vi "Camera To Target Grid.vi"(2 "Height":dbl format="%#_13g", 3 "Width":dbl format="%#_13g", 4 "CY":dbl format="%#_13g", 5 "CX":dbl format="%#_13g") -> (0 "Y'":dbl format="%#_13g", 1 "X'":dbl format="%#_13g")   [LabVIEW 2013]
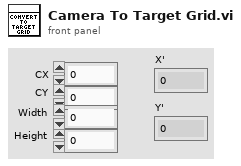
[diagram p1: front panel]
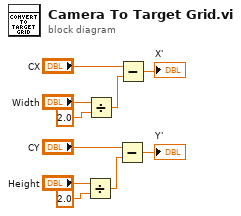
[diagram p0: block diagram]
diagram:
  n1 = Divide(x="Height", y=2.0) -> (x/y=w4:dbl)
  n2 = Divide(x="Width", y=2.0) -> (x/y=w8:dbl)
  n3 = Subtract(x="CY", y=w4) -> (x-y=→"Y'":dbl)
  n4 = Subtract(x="CX", y=w8) -> (x-y=→"X'":dbl)
